vi "Fetch Multi-Point [MP] Core.vi"(8 "error in (no error)":errorcluster, 9 "array size":i32, 10 "maximum time (5s)":dbl[unit]=5000.0 caption="maximum time (5000 ms)", 11 "IVI_DMM in":refnum<class "IVI_DMM.lvclass">) -> (0 "error out":errorcluster, 1 "actual number of points":i32, 2 "reading array":dbl[](array[numeric]) format="%^.2e", 3 "IVI_DMM out":refnum<class "IVI_DMM.lvclass">)   [LabVIEW 2013, in "IVI_DMM.lvlib" / "IVI_DMM.lvclass"]
doc: "This VI returns an array of values from a previously initiated multi-point measurement. The number of measurements the DMM takes is determined by the values you specify for the Trigger Count and Sample Count parameters of the IviDmm Configure Multi-Point [MP] VI.\n\nYou must first call the IviDmm Initiate VI to initiate a measurement before calling this VI.\n\nNotes:\n\n(1) This VI is part of the IviDmmMultiPoint [MP] extension group.\n\n(2) After this VI executes, each element in the Reading Array parameter is an actual reading or a value indicating that an over-range condition occurred.\n\n(3) If an over-range condition occurs, the corresponding Reading Array element contains an IEEE defined NaN (Not a Number) value and the VI returns IVIDMM_WARN_OVER_RANGE (0x3FFA2001). \n\n(4) You can test each element in the Reading Array parameter for over-range with the IviDmm Is Over-Range VI.\n\n(5) The class driver returns a simulated measurement when this VI is called and the IviDmm>>Inherent IVI Settings>>User Options>>Simulate property is set to TRUE and the IviDmm>>Inherent IVI Settings>>User Options>>Use Specific Simulation property is set to FALSE. For information on how to configure a simulated measurement, refer to the online help manual.\n\n(6) This VI does not check the instrument status. Typically, you call this VI only in a sequence of calls to other low-level driver VIs. The sequence performs one operation. You use the low-level VIs to optimize one or more aspects of interaction with the instrument. If you want to check the instrument status, call the IviDmm Error-Query VI at the conclusion of the sequence."
uses:
  IVI_DMM.lvclass
  IVI_DMM.lvclass/IVI_DMM.ctl
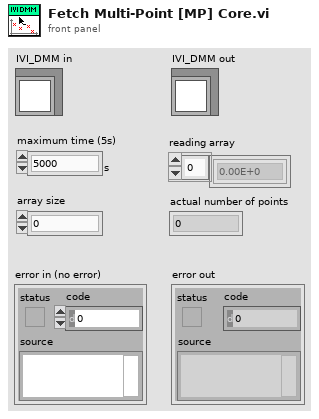
[diagram p1: front panel]
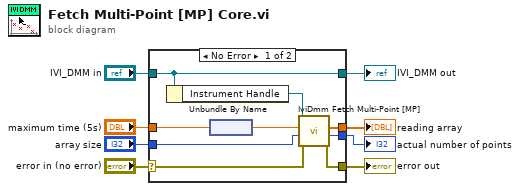
[diagram p0: block diagram]
diagram:
  n1 = case shown="No Error" "error in (no error)" {
    selector: "error in (no error)" -> [w15 w19]
    tunnel: [w14 w19] -> w1
    tunnel: [w17 w18] -> w2
    tunnel: "IVI_DMM in" -> [w17 w18]
    tunnel: "maximum time (5s)" -> [w13 _]
    tunnel: "array size" -> [w11 _]
    tunnel: [w10 _] -> w4
    tunnel: [w9 _] -> w3
    frame No Error {
      n2 = Unbundle By Name(w17) -> ("Instrument Handle"=w16:refnum<k15>)
      n3 = node(w13) -> (w12:dbl)
      n4 = call <vilib>:"IviDmm Fetch Multi-Point [MP].vi"("error in (no error)"=w15, "array size (1)"=w11, "maximum time (5000 ms)"=w12, "instrument handle"=w16) -> ("error out"=w14:errorcluster, "actual number of points"=w9:i32, "reading array"=w10:dbl[])  [unwired: 4 in, 1 out]
    }
    frame Error {
    }
  }
  "error out" <- w1
  "IVI_DMM out" <- w2
  "reading array" <- w4
  "actual number of points" <- w3
